vi "getNumber.vi"(8 "error in (no error)":errorcluster, 11 "Tab Control":refnum<vi>) -> (0 "error out":errorcluster, 2 "Number":dbl)   [LabVIEW 2011, in "Views.lvlib" / "Camera.lvlib" / "andorSettingsViewer.lvclass"]
uses:
  andorSettingsViewer.lvclass
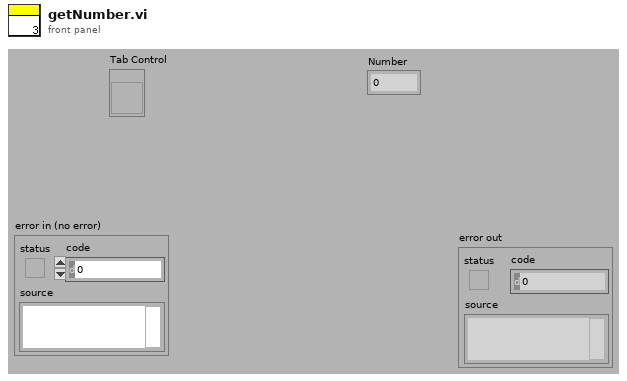
[diagram p1: front panel]
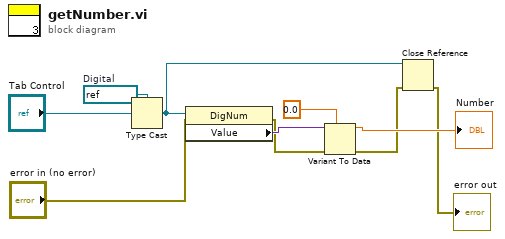
[diagram p0: block diagram]
diagram:
  w10 = refnum<vi> refnum  # Digital
  n1 = Type Cast(type=w10, x="Tab Control") -> (*(type *) &x=w1:refnum<vi>)
  n2 = property class="DigNum"(reference=w1, error in="error in (no error)") -> (error out=w7:errorcluster, "Value"=w8:variant)  [unwired: 1 out]
  n3 = Variant To Data(error in=w7, type=0.0, Variant=w8) -> (data=→"Number":dbl, error out=w3:errorcluster)
  n4 = Close Reference(reference=w1, error in (no error)=w3) -> (error out=→"error out":errorcluster)
